vi "Flashing_binary_Test.vi"() -> ()   [LabVIEW 2017]
panel:
  out "String":string
  out "%":dbl
  out "Flashing SC/AC/PC inprogress......":u8(slide) scale=0.0..100.0
  out "FW Upgrade bytes":string
  out "Test Result":picture
  # "FLASHING BINARY TO ULTRASONIC WELDING MACHINE\nSC/AC/PC"
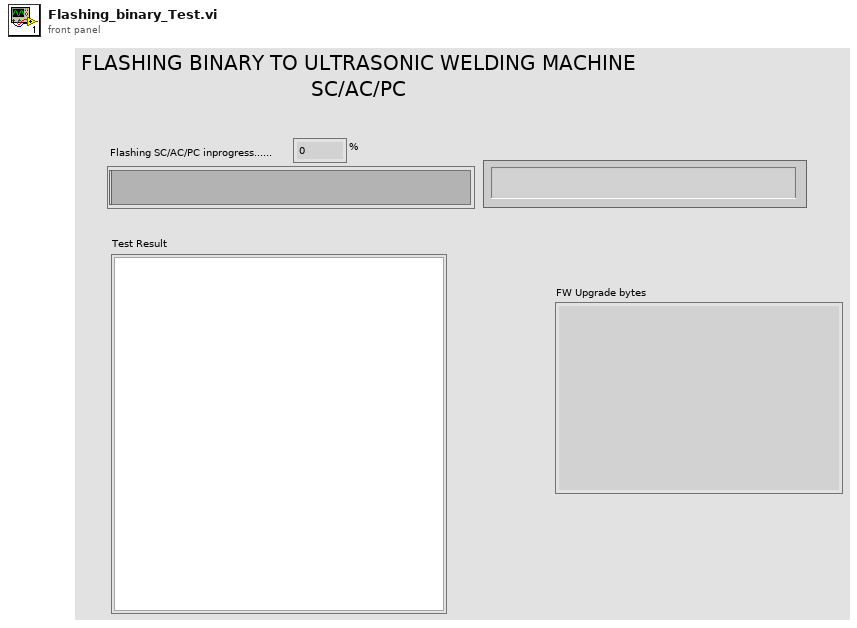
[diagram p1: front panel]
types:
  T1 = enum16{"open", "replace", "create", "open or create", "replace or create", "replace or create with confirmation"}
  T2 = cluster{"[0]":string, "[1]":string, "[2]":string, "[3]":string, "[4]":string, "[5]":string, "[6]":string, "[7]":string, "[8]":string}
  T3 = cluster{"Iterations":u64, "DelayBetweenIterations":u32, "Timeout":u32, "MessageID":i32, "MessageLength":i32, "ResponseID":i32, "AC_PC_SC":string, "Timestamp":string, "TestSuite":string, "ReportPath":path, "FWVersionPath":path}
  T4 = cluster{"Socket_IP_Address":string, "Socket_Port_Number":u16, "Global_ReportPath":path}
  T5 = typedef "imagedata.ctl" = cluster{"image type":i32, "image depth":i32, "image":u8[], "mask":u8[], "colors":u32[], "Rectangle":cluster{"left":i16, "top":i16, "right":i16, "bottom":i16}}
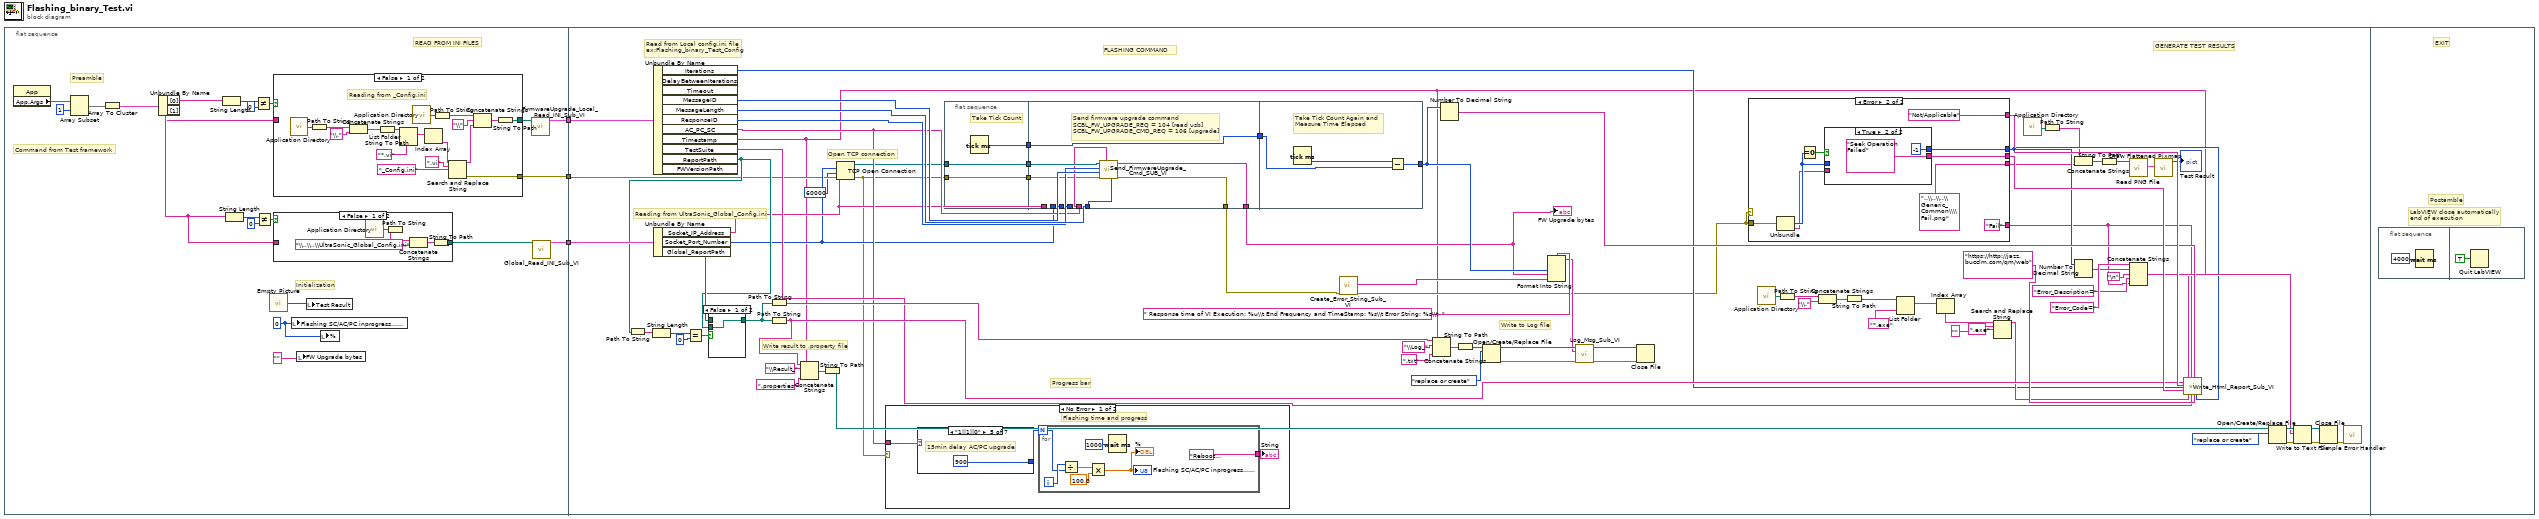
[diagram p0: block diagram]
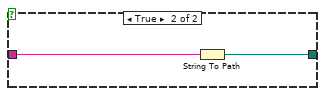
[diagram p2: hidden frame]
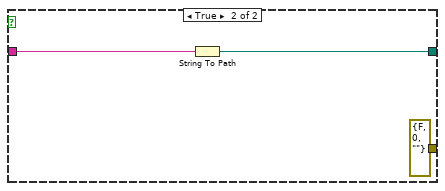
[diagram p3: hidden frame]
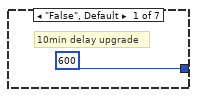
[diagram p4: hidden frame]
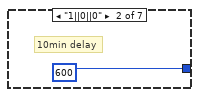
[diagram p5: hidden frame]
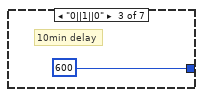
[diagram p6: hidden frame]
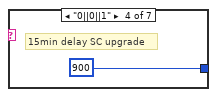
[diagram p7: hidden frame]
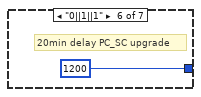
[diagram p8: hidden frame]
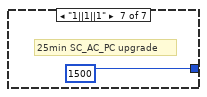
[diagram p9: hidden frame]
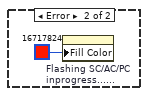
[diagram p10: hidden frame]
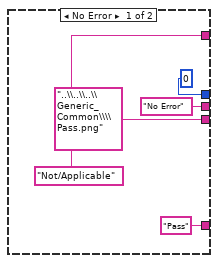
[diagram p12: hidden frame]
diagram:
  n1 = flat-sequence {
    tunnel: [w9] -> w3
    tunnel: [w8] -> w2
    tunnel: [w7] -> w1
    tunnel: w3 -> [w60]
    tunnel: w2 -> [w78]
    tunnel: w1 -> [w75]
    frame #0 {
      w5 = 0
      # "READ FROM INI FILES"
      # "Command from Test framework"
      # "Initialization"
      # "Preamble"
      n2 = property class="App"() -> ("App.Args"=w11:string[])  [unwired: 2 in, 2 out]
      n3 = Array Subset "Array Subset"(array=w11, index=1) -> (w12:string[])  [unwired: 1 in]
      n4 = Array To Cluster(array=w12) -> (cluster=w13:T2)
      n5 = Unbundle By Name "Unbundle By Name"(w13) -> ("[0]"=w17:string, "[1]"=w20:string)
      n6 = String Length(string=w17) -> (length=w14:i32)
      n7 = String Length(string=w20) -> (length=w21:i32)
      n8 = Not Equal?(x=w14, y=0) -> (x != y?=w16:bool)
      n9 = Not Equal?(x=w21, y=0) -> (x != y?=w19:bool)
      n10 = call "Empty Picture"() -> ("empty picture"=w6:picture)
      n11 = case shown="False" w16 {
        tunnel: w17 -> [_ w50]
        tunnel: [w32 w49] -> w22
        tunnel: [w31 errorcluster {"status"=FALSE, "code"=0, "source"=""} ("error out")] -> w9
        frame False {
          # "Reading from _Config.ini"
          n12 = call <vilib>:"Application Directory.vi"() -> ("Application Directory"=w38:path)
          n13 = Path To String(path=w38) -> (string=w37:string)
          n14 = Concatenate Strings(w37, "\\." ("string")) -> (w35:string)
          n15 = String To Path(string=w35) -> (path=w40:path)
          n16 = List Folder(path=w40, pattern="*.vi") -> (filenames=w34:string[])  [unwired: 2 in, 3 out]
          n17 = call <vilib>:"Application Directory.vi"() -> ("Application Directory"=w47:path)
          n18 = Index Array(array=w34) -> (element=w33:string)  [unwired: 1 in]
          n19 = Path To String(path=w47) -> (string=w42:string)
          n20 = Search and Replace String(input string=w33, search string=".vi", replace string="_Config.ini" ("replace string (\"\")")) -> (result string=w44:string, error out=w31:errorcluster)  [unwired: 5 in, 2 out]
          n21 = Concatenate Strings(w42, "\\" ("string"), w44) -> (w41:string)
          n22 = String To Path(string=w41) -> (path=w32:path)
        }
        frame True {
          n23 = String To Path(string=w50) -> (path=w49:path)
        }
      }
      n24 = case shown="False" w19 {
        tunnel: [w25 w30] -> w23
        tunnel: w20 -> [_ w29]
        frame False {
          n25 = call <vilib>:"Application Directory.vi"() -> ("Application Directory"=w24:path)
          n26 = Path To String(path=w24) -> (string=w28:string)
          n27 = Concatenate Strings(w28, "\\..\\..\\UltraSonic_Global_Config.ini" ("string")) -> (w26:string)
          n28 = String To Path(string=w26) -> (path=w25:path)
        }
        frame True {
          n29 = String To Path(string=w29) -> (path=w30:path)
        }
      }
      n30 = local write "Flashing SC/AC/PC inprogress......"(w5) -> ()
      n31 = local write "FW Upgrade bytes"("") -> ()
      n32 = local write "Test Result"(w6) -> ()
      n33 = local write "%"(w5) -> ()
      n34 = call "FirmwareUpgrade_Local_Read_INI_Sub_VI.vi"("Config File Path"=w22) -> ("output"=w7:T3)  [unwired: 10 in]
      n35 = call "Global_Read_INI_Sub_VI.vi"("Config File Path"=w23) -> ("output cluster"=w8:T4)  [unwired: 14 in]
    }
    frame #1 {
      # "GENERATE TEST RESULTS"
      # "FLASHING COMMAND"
      # "Progress bar"
      # "Write to Log file"
      # "Write result to .property file"
      # "Open TCP connection"
      # "Read from Local config.ini file\nex:Flashing_binary_Test_Config"
      # "Reading from UltraSonic_Global_Config.ini"
      n36 = Unbundle By Name(w75) -> ("Iterations"=w76:u64, "MessageID"=w74:i32, "MessageLength"=w73:i32, "ResponseID"=w72:i32, "AC_PC_SC"=w69:string, "Timestamp"=w51:string, "TestSuite"=w71:string, "ReportPath"=w70:path)  [unwired: 3 out]
      n37 = Path To String(path=w70) -> (string=w124:string)
      n38 = String Length(string=w124) -> (length=w123:i32)
      n39 = Unbundle By Name(w78) -> ("Socket_IP_Address"=w62:string, "Socket_Port_Number"=w61:u16, "Global_ReportPath"=w77:path)
      n40 = Equal?(x=w123, y=0) -> (x = y?=w121:bool)
      n41 = case shown="False" w121 {
        tunnel: w77 -> [_ w168]
        tunnel: [w167 w168] -> w120
        tunnel: w70 -> [w167 _]
        frame False {
        }
        frame True {
        }
      }
      n42 = Path To String(path=w120) -> (string=w126:string)
      n43 = Path To String(path=w120) -> (string=w97:string)
      n44 = Concatenate Strings(w97, "\\Result_" ("string"), w51, ".properties" ("string")) -> (w118:string)
      n45 = String To Path(string=w118) -> (path=w110:path)
      n46 = TCP Open Connection(address=w62, remote port or service name=w61, timeout ms (60000)=60000, error in (no error)=w60) -> (connection ID=w57:refnum<k5>, error out=w55:errorcluster)  [unwired: 1 in]
      n47 = case shown="No Error" w55 {
        tunnel: w69 -> [w151 _]
        frame No Error {
          # "Flashing time and progress"
          n48 = case shown="\"1||1||0\"" w151 {
            tunnel: [600 600 600 900 900 1200 1500] -> w150
            frame "False", Default {
              # "10min delay upgrade"
            }
            frame "1||0||0" {
              # "10min delay"
            }
            frame "0||1||0" {
              # "10min delay"
            }
            frame "0||0||1" {
              # "15min delay SC upgrade"
            }
            frame "1||1||0" {
              # "15min delay AC/PC upgrade"
            }
            frame "0||1||1" {
              # "20min delay PC_SC upgrade"
            }
            frame "1||1||1" {
              # "25min SC_AC_PC upgrade"
            }
          }
          n49 = for {
            N: w150 -> [w156]
            tunnel: ["Reboot the system flashing is completed...!!!"] -> w149
            i -> [w157]
            n50 = Divide(x=w157, y=w156) -> (x/y=w155:dbl)
            n51 = Multiply(x=w155, y=100.0) -> (x*y=→"Flashing SC/AC/PC inprogress......" →"%":dbl)
            n52 = Wait (ms)(milliseconds to wait=u32 1000) -> ()  [unwired: 1 out]
          }
          "String" <- w149
        }
        frame Error {
          n53 = property on="Flashing SC/AC/PC inprogress......" class="Slide (strict)"("Fill Color"=u32 16717824) -> ()  [unwired: 2 in, 2 out]
        }
      }
      n54 = flat-sequence {
        tunnel: [w136] -> w68
        tunnel: [w135] -> w58
        tunnel: w57 -> [w135]
        tunnel: [w134] -> w56
        tunnel: w55 -> [w134]
        tunnel: [w145] -> w67
        tunnel: w68 -> [w145]
        tunnel: w62 -> [_]
        tunnel: w61 -> [_]
        tunnel: w74 -> [w144]
        tunnel: w73 -> [w143]
        tunnel: w72 -> [w142]
        tunnel: w69 -> [w140]
        tunnel: w58 -> [w141]
        tunnel: w56 -> [w139]
        tunnel: [w138] -> w54
        tunnel: [w137] -> w52
        tunnel: w67 -> [w148]
        tunnel: [w146] -> w64
        frame #0 {
          # "Take Tick Count"
          n55 = Tick Count (ms)() -> (millisecond timer value=w136:u32)
        }
        frame #1 {
          # "Send firmware upgrade command \nSCBL_FW_UPGRADE_REQ = 104 [read usb]\nSCBL_FW_UPGRADE_CMD_REQ = 106 [upgrade]"
          n56 = call "Send_FirmwareUpgrade_Cmd_SUB_VI.vi"("Message Length"=w143, "Which one to upgrade? AC||PC||SC"=w140, "Error Input"=w139, "Message ID"=w144, "Response ID"=w142, "TCP_IN"=w141) -> ("Error Out put"=w138:errorcluster, "FW Upgrade Results"=w137:string)  [unwired: 4 in]
        }
        frame #2 {
          # "Take Tick Count Again and Measure Time Elapsed"
          n57 = Tick Count (ms)() -> (millisecond timer value=w147:u32)
          n58 = Subtract(x=w147, y=w148) -> (x-y=w146:u32)
        }
      }
      n59 = call "Create_Error_String_Sub_VI.vi"("error in"=w54) -> ("error out"=w53:errorcluster, "Error String"=w63:string)  [unwired: 9 in]
      n60 = Concatenate Strings(w126, "\\Log_" ("string"), w51, ".txt" ("string")) -> (w129:string)
      n61 = Number To Decimal String(number=w64) -> (decimal integer string=w131:string)  [unwired: 1 in]
      n62 = String To Path(string=w129) -> (path=w128:path)
      n63 = Open/Create/Replace File(file path (use dialog)=w128, operation (0:open)=T1."replace or create") -> (refnum out=w98:refnum<file>, error out=w101:errorcluster)  [unwired: 1 in, 4 out]
      n64 = Format Into String(format string=" Response time of VI Execution: %u\\t End Frequency and TimeStamp: %s\\t Error String: %s\\t  ", w64, w52, w63) -> (resulting string=w65:string)  [unwired: 2 in, 1 out]
      n65 = call "Log_Msg_Sub_VI.vi"("error in (no error)"=w101, "String"=w65, "Byte Stream File in"=w98) -> ("error out"=w99:errorcluster, "Byte Stream File out"=w100:refnum<file>)  [unwired: 7 in]
      n66 = Close File(refnum=w100, error in=w99) -> ()  [unwired: 2 out]
      n67 = case shown="Error" w53 {
        tunnel: ["Pass" "Fail"] -> w102
        tunnel: w53 -> [_ w180]
        tunnel: [0 ("code") w176] -> w106
        tunnel: ["No Error" ("source") w177] -> w133
        tunnel: ["Not/Applicable" "Not/Applicable"] -> w132
        tunnel: ["..\\..\\..\\Generic_Common\\\\Pass.png" ("string") "..\\..\\..\\Generic_Common\\\\Fail.png" ("string")] -> w79
        frame No Error {
        }
        frame Error {
          n68 = Unbundle(w180) -> ("code"=w178:i32, "source"=w174:string)  [unwired: 1 out]
          n69 = Equal To 0?(x=w178) -> (x = 0?=w175:bool)
          n70 = case shown="True" w175 {
            tunnel: [w184 -1 ("code")] -> w176
            tunnel: [w183 "Seek Operation Failed" ("source")] -> w177
            tunnel: w178 -> [w184 _]
            tunnel: w174 -> [w183 _]
            frame False {
            }
            frame True {
            }
          }
        }
      }
      n71 = call <vilib>:"Application Directory.vi"() -> ("Application Directory"=w94:path)
      n72 = Path To String(path=w94) -> (string=w93:string)
      n73 = Concatenate Strings(w93, "\\." ("string")) -> (w91:string)
      n74 = String To Path(string=w91) -> (path=w96:path)
      n75 = List Folder(path=w96, pattern="*.exe") -> (filenames=w90:string[])  [unwired: 2 in, 3 out]
      n76 = Index Array(array=w90) -> (element=w86:string)  [unwired: 1 in]
      n77 = Search and Replace String(input string=w86, search string=".exe", replace string="" ("replace string (\"\")")) -> (result string=w89:string)  [unwired: 5 in, 3 out]
      n78 = call <vilib>:"Application Directory.vi"() -> ("Application Directory"=w80:path)
      n79 = Path To String(path=w80) -> (string=w81:string)
      n80 = Concatenate Strings(w81, w79) -> (w82:string)
      n81 = Number To Decimal String(number=w106) -> (decimal integer string=w105:string)  [unwired: 1 in]
      n82 = String To Path(string=w82) -> (path=w85:path)
      n83 = call <vilib>:"Read PNG File.vi"("path to PNG file"=w85) -> ("image data"=w83:T5)  [unwired: 8 in, 2 out]
      n84 = Concatenate Strings("Error_Code=" ("string"), w105, "\n", "Error_Description=" ("string"), w102) -> (w108:string)
      n85 = call <vilib>:"Draw Flattened Pixmap.vi"("image data"=w83) -> ("new picture"=→"Test Result":picture)  [unwired: 8 in]
      n86 = call "Write_Html_Report_Sub_VI.vi"("ReprtPath"=w97, "Remarks"=w132, "Iterations"=w76, "Error Description"=w133, "Timestamp"=w51, "TestCase"=w89, "Verdict"=w102, "TestSuite"=w71, "Time taken to execute  test in msec"=w131, "JazzDashboardLink"="https://http://jazz.bucclm.com/qm/web" ("TestSuite"), "Error Code"=w106) -> ()  [unwired: 9 in]
      n87 = Open/Create/Replace File(file path (use dialog)=w110, operation (0:open)=T1."replace or create") -> (refnum out=w109:refnum<file>, error out=w114:errorcluster)  [unwired: 4 in, 1 out]
      n88 = Write to Text File(file (use dialog)=w109, text=w108, error in=w114) -> (refnum out=w113:refnum<file>, error out=w112:errorcluster)  [unwired: 1 in, 1 out]
      n89 = Close File(refnum=w113, error in=w112) -> (error out=w111:errorcluster)  [unwired: 1 out]
      n90 = call <vilib>:"Simple Error Handler.vi"("error in (no error)"=w111) -> ()  [unwired: 4 in, 5 out]
      "FW Upgrade bytes" <- w52
    }
    frame #2 {
      # "EXIT"
      # "LabVIEW close automatically \nend of execution"
      # "Postamble"
      n91 = flat-sequence {
        frame #0 {
          n92 = Wait (ms)(milliseconds to wait=u32 4000) -> ()  [unwired: 1 out]
        }
        frame #1 {
          n93 = Quit LabVIEW(quit? (T)=TRUE) -> ()
        }
      }
    }
  }
